vi "RW_Module.vi"(7 "N_moduls":i32, 8 "error in":errorcluster, 9 "Param Referense":T1, 10 "Data Reference":T2, 11 "Status Reference":T3) -> (0 "error out":errorcluster, 1 "stopped":bool)   [LabVIEW 2019]
uses:
  Eth Status/Ctl/ICPCON Status.ctl
  MB_TCP_State.ctl
  ICPCON Registers/Ctl/ICPCON Data.ctl
  ICPCON Param/ICPCON Param.ctl
  ICPCON Param/Eth timeouts.ctl
  ICPCON ET-7018/ICPCON ET-7018.lvclass
  D:/my_projects/projects/Algorithms/Labview/19/Modbus/MB_TCP2/MB_TCP.lvclass
  ICPCON ET-7016/ICPCON ET-7016.lvclass
  ICPCON ET-7051/ICPCON ET-7051.lvclass
  ICPCON ET-7017/ICPCON ET-7017.lvclass
  ICPCON ET-7018i/ICPCON ET-7018i.lvclass
  ICPCON ET-7024i/ICPCON ET-7024i.lvclass
  ZERO/ZERO.lvclass
  NS300/NS300.lvclass
  ICPCON ET-7042i/ICPCON ET-7042i.lvclass
  TEST/TEST.lvclass
  LIR-919D/LIR-919D.lvclass
  ICPCON ET-7016i/ICPCON ET-7016i.lvclass
  ICPCON ET-7024/ICPCON ET-7024.lvclass
  SMSD/SMSD-AI/SMSD-AI.lvclass
  SMSD/SMSD-DI/SMSD-DI.lvclass
  MB timeouts.ctl
  NI_modbus_upd/TCP/tcp timeouts.ctl
  MB_TCP.lvclass/MB_TCP.ctl
  NI_modbus_upd/TCP/TCP.lvclass/TCP.ctl
  Execute.vi
  MB_TCP.lvclass
  Eth Status/Eth Status.lvlib
  ICPCON Param/ICPCON_Param.lvlib
  NI_modbus_upd/TCP/TCP.lvclass
  ICPCON Registers/ICPCON Registers.lvlib
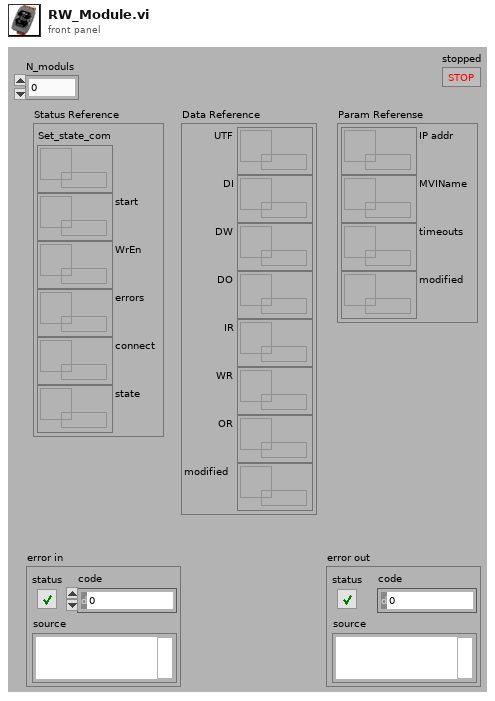
[diagram p1: front panel]
types:
  T1 = typedef "ICPCON_Param.lvlib/ICPCON Param.ctl" = cluster{"IP addr":refnum<data-value>, "MVIName":refnum<data-value>, "timeouts":refnum<data-value>, "modified":refnum<data-value>}
  T2 = typedef "ICPCON Registers.lvlib/ICPCON Data.ctl" = cluster{"UTF":refnum<data-value>, "DI":refnum<data-value>, "DW":refnum<data-value>, "DO":refnum<data-value>, "IR":refnum<data-value>, "WR":refnum<data-value>, "OR":refnum<data-value>, "modified":refnum<data-value>}
  T3 = typedef "Eth Status.lvlib/ICPCON Status.ctl" = cluster{"Set_state_com":refnum<data-value>, "start":refnum<data-value>, "WrEn":refnum<data-value>, "errors":refnum<data-value>, "connect":refnum<data-value>, "state":refnum<data-value>}
  T4 = enum16{"initialize", "call modules", "work", "stop modules", "standby"}
  T5 = typedef "TCP.lvclass/tcp timeouts.ctl" = cluster{"connect timeout":i32, "write timeout":i32, "read timeout":i32}
  T6 = typedef "MB_TCP.lvclass/MB timeouts.ctl" = cluster{"reconn_timeout":i32, "N attempt max":i32, "t_reset_TTL":i32, "period":i32}
  T7 = typedef "ICPCON_Param.lvlib/Eth timeouts.ctl" = cluster{"conn_timeout":i32, "reconn_timeout":i32, "N attempt max":i32, "t_reset_TTL":i32, "write_timeout":i32, "read_timeout":i32, "period":i32}
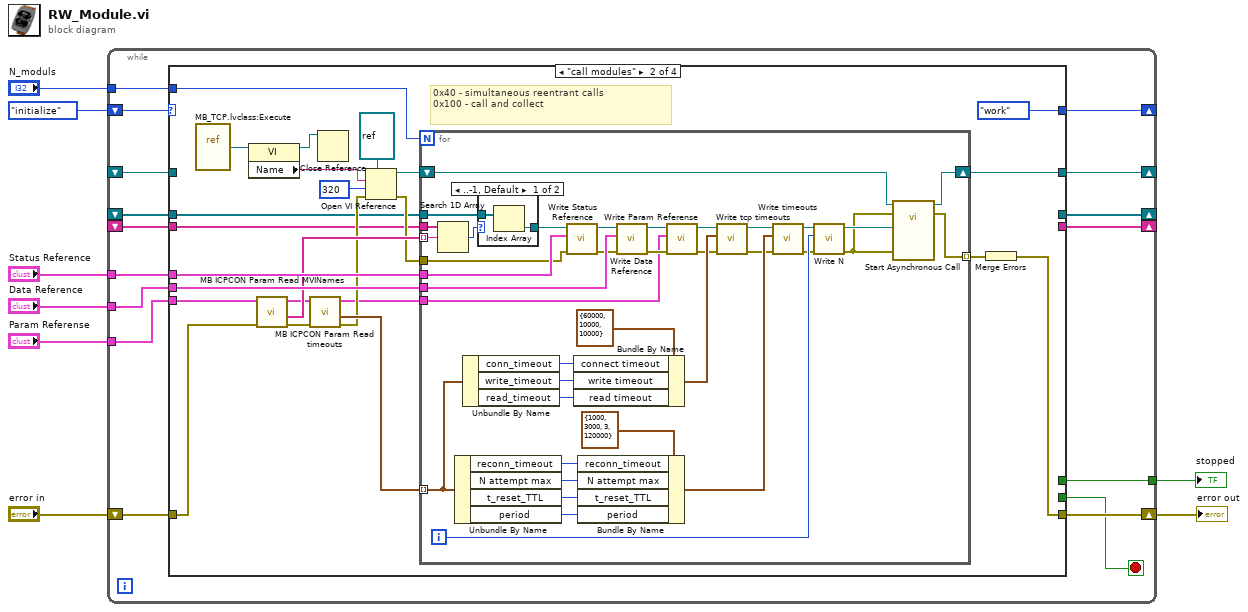
[diagram p0: block diagram]
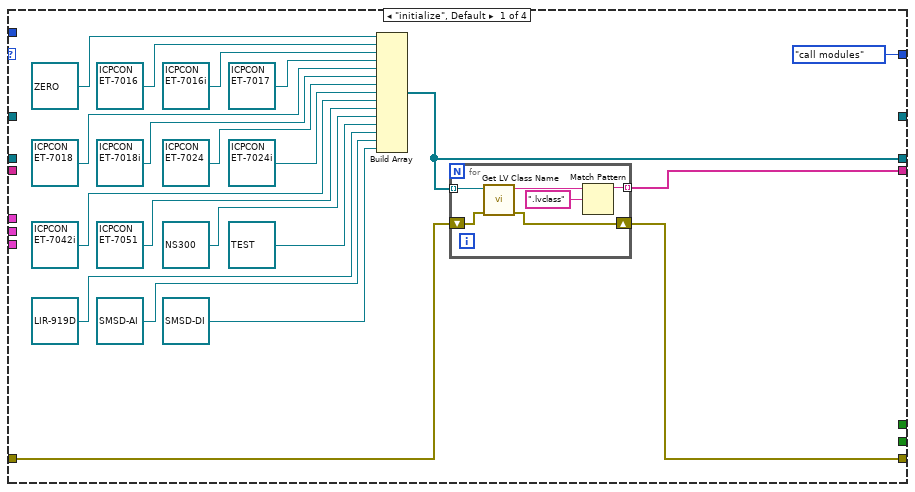
[diagram p2: hidden frame]
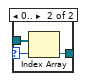
[diagram p3: hidden frame]
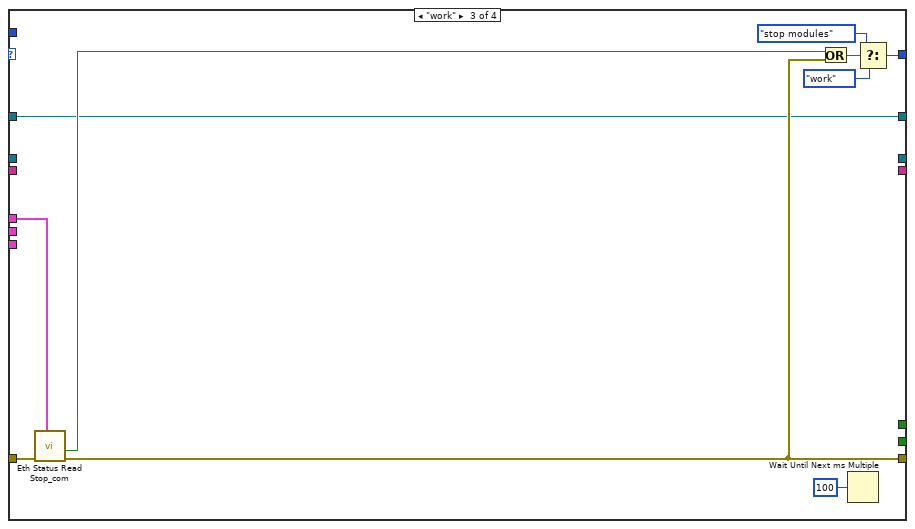
[diagram p4: hidden frame]
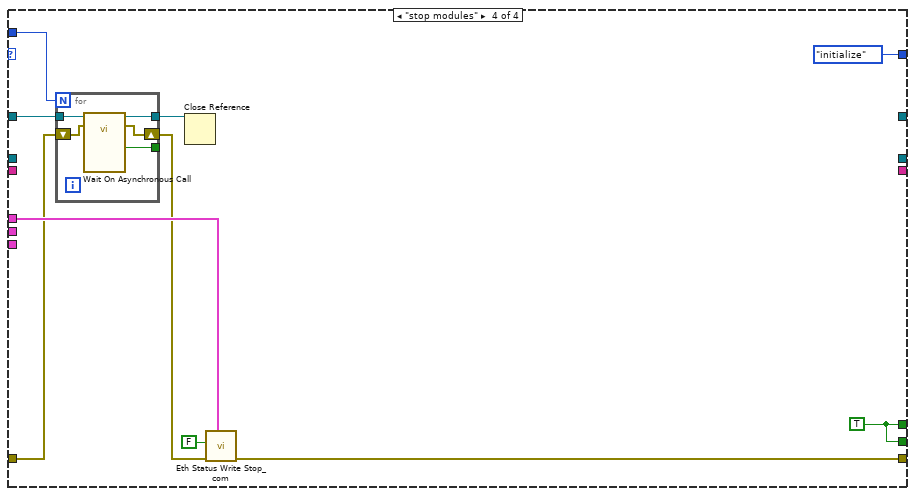
[diagram p5: hidden frame]
diagram:
  n1 = while {
    shift-right: [w24] -> _
    shift-left: T4."initialize" ("Enum") -> [w23]
    shift-right: [w22] -> w7
    shift-left: "error in" -> [w21]
    tunnel: [w20] -> w6
    tunnel: "Param Referense" -> [w18]
    tunnel: "Data Reference" -> [w17]
    tunnel: "Status Reference" -> [w16]
    tunnel: "N_moduls" -> [w15]
    shift-right: [w14] -> _
    shift-left: _ -> [w13]
    shift-right: [w12] -> _
    shift-left: _ -> [w10]
    shift-right: [w11] -> _
    shift-left: _ -> [w9]
    stop <- w19 stop-if-true
    n2 = case shown="\"call modules\"" w23 {
      tunnel: [T4."call modules" ("Enum") T4."work" ("Enum") w126 T4."initialize" ("Enum")] -> w24
      tunnel: w15 -> [_ w66 _ w127]
      tunnel: w16 -> [_ w73 w120 w134]
      tunnel: [w42 w72 w118 w133] -> w22
      tunnel: w21 -> [w43 w54 w121 w130]
      tunnel: [_ _ _ w136] -> w20
      tunnel: [_ _ _ w136] -> w19
      tunnel: w17 -> [_ w69 _ _]
      tunnel: w18 -> [_ w53 _ _]
      tunnel: [_ w57 w117 _] -> w14
      tunnel: w13 -> [_ _ w117 w131]
      tunnel: [w41 _ _ _] -> w12
      tunnel: [w40 _ _ _] -> w11
      tunnel: w10 -> [_ w56 _ _]
      tunnel: w9 -> [_ w55 _ _]
      frame "initialize", Default {
        n3 = Build Array(refnum<class "ZERO.lvclass"> refnum ("ZERO.lvclass"), refnum<class "ICPCON ET-7016.lvclass"> refnum ("ICPCON ET-7016.lvclass"), refnum<class "ICPCON ET-7016i.lvclass"> refnum ("ICPCON ET-7016i.lvclass"), refnum<class "ICPCON ET-7017.lvclass"> refnum ("ICPCON ET-7017.lvclass"), refnum<class "ICPCON ET-7018.lvclass"> refnum ("ICPCON ET-7018 in"), refnum<class "ICPCON ET-7018i.lvclass"> refnum ("ICPCON ET-7018i.lvclass"), refnum<class "ICPCON ET-7024.lvclass"> refnum ("ICPCON ET-7024.lvclass"), refnum<class "ICPCON ET-7024i.lvclass"> refnum ("ICPCON ET-7024i.lvclass"), refnum<class "ICPCON ET-7042i.lvclass"> refnum ("ICPCON ET-7042i.lvclass"), refnum<class "ICPCON ET-7051.lvclass"> refnum ("ICPCON ET-7051.lvclass"), refnum<class "NS300.lvclass"> refnum ("NS300.lvclass"), refnum<class "TEST.lvclass"> refnum ("TEST.lvclass"), refnum<class "LIR-919D.lvclass"> refnum ("LIR-919D.lvclass"), refnum<class "SMSD-AI.lvclass"> refnum ("SMSD-AI.lvclass"), refnum<class "SMSD-DI.lvclass"> refnum ("SMSD-DI.lvclass")) -> (w41:refnum<class "MB_TCP.lvclass">[])
        n4 = for {
          tunnel: w41 -> [w50] mode=indexing
          tunnel: [w46] -> w40 mode=indexing
          shift-right: [w49] -> w42
          shift-left: w43 -> [w45]
          n5 = call <vilib>:"Get LV Class Name.vi"("error in (no error)"=w45, "object"=w50) -> ("error out"=w49:errorcluster, "class name"=w48:string)  [unwired: 8 in]
          n6 = Match Pattern(string=w48, regular expression=".lvclass") -> (before substring=w46:string)  [unwired: 1 in, 3 out]
        }
      }
      frame "call modules" {
        # "0x40 - simultaneous reentrant calls\n0x100 - call and collect"
        n7 = vi-ref "MB_TCP.lvclass:Execute.vi"() -> (w70:refnum<vi>)
        n8 = property class="VI"(reference=w70) -> (reference out=w64:refnum<vi>, "Name"=w61:string)  [unwired: 1 in, 1 out]
        n9 = call "MB ICPCON Param Read MVINames.vi"("error in (no error)"=w54, "Param Reference in"=w53) -> ("error out"=w65:errorcluster, "MVIName"=w67:string[], "Param Reference out"=w52:T1)  [unwired: 7 in]
        n10 = call "MB ICPCON Param Read timeouts.vi"("error in (no error)"=w65, "Param Reference in"=w52) -> ("error out"=w62:errorcluster, "timeouts"=w68:T7[], "Param Reference out"=w51:T1)  [unwired: 7 in]
        n11 = Close Reference(reference=w64) -> ()  [unwired: 1 in, 1 out]
        n12 = Open VI Reference(type specifier VI Refnum (for type only)=refnum<vi> refnum, vi path=w61, options=320, error in (no error)=w62) -> (vi reference=w59:refnum<vi>, error out=w60:errorcluster)  [unwired: 2 in]
        n13 = for {
          N: w66 -> [_]
          tunnel: [w111] -> w74 mode=indexing
          tunnel: w68 -> [w81] mode=indexing
          tunnel: w67 -> [w97] mode=indexing
          tunnel: w73 -> [w108]
          tunnel: w69 -> [w107]
          tunnel: w56 -> [w110]
          tunnel: w55 -> [w109]
          tunnel: w60 -> [w96]
          shift-right: [w94] -> w57
          shift-left: w59 -> [w95]
          tunnel: w51 -> [w86]
          i -> [w99]
          n14 = Search 1D Array(1D array=w109, element=w97) -> (index of element=w106:i32)  [unwired: 1 in]
          n15 = Unbundle By Name(w81) -> ("reconn_timeout"=w104:i32, "N attempt max"=w103:i32, "t_reset_TTL"=w102:i32, "period"=w101:i32)
          n16 = Unbundle By Name(w81) -> ("conn_timeout"=w84:i32, "write_timeout"=w83:i32, "read_timeout"=w82:i32)
          n17 = case shown="..-1, Default" w106 {
            selector: w106 -> [_ w114]
            tunnel: w110 -> [w113 w116]
            tunnel: [w112 w115] -> w98
            frame ..-1, Default {
              n18 = Index Array(array=w113) -> (element=w112:refnum<class "MB_TCP.lvclass">)  [unwired: 1 in]
            }
            frame 0.. {
              n19 = Index Array(array=w116, index=w114) -> (element=w115:refnum<class "MB_TCP.lvclass">)
            }
          }
          n20 = call "Write Status Reference.vi"("error in (no error)"=w96, "Status"=w108, "MB_TCP in"=w98) -> ("error out"=w89:errorcluster, "MB_TCP out"=w90:refnum<class "MB_TCP.lvclass">)  [unwired: 7 in]
          n21 = Bundle By Name(cluster=T5 {"connect timeout"=60000, "write timeout"=10000, "read timeout"=10000} ("tcp timeouts"), "connect timeout"=w84, "write timeout"=w83, "read timeout"=w82) -> (w80:T5)
          n22 = Bundle By Name(cluster=T6 {"reconn_timeout"=1000, "N attempt max"=3000, "t_reset_TTL"=3, "period"=120000} ("timeouts"), "reconn_timeout"=w104, "N attempt max"=w103, "t_reset_TTL"=w102, "period"=w101) -> (w100:T6)
          n23 = call "Write Data Reference.vi"("error in (no error)"=w89, "Data"=w107, "MB_TCP in"=w90) -> ("error out"=w87:errorcluster, "MB_TCP out"=w88:refnum<class "MB_TCP.lvclass">)  [unwired: 7 in]
          n24 = call "Write Param Referense.vi"("error in (no error)"=w87, "Param Referense"=w86, "MB_TCP in"=w88) -> ("error out"=w78:errorcluster, "MB_TCP out"=w79:refnum<class "MB_TCP.lvclass">)  [unwired: 7 in]
          n25 = call "Write tcp timeouts.vi"("error in (no error)"=w78, "tcp timeouts"=w80, "MB_TCP in"=w79) -> ("error out"=w76:errorcluster, "MB_TCP out"=w77:refnum<class "MB_TCP.lvclass">)  [unwired: 7 in]
          n26 = call "Write timeouts.vi"("error in (no error)"=w76, "MB timeouts"=w100, "MB_TCP in"=w77) -> ("error out"=w92:errorcluster, "MB_TCP out"=w91:refnum<class "MB_TCP.lvclass">)  [unwired: 7 in]
          n27 = call "Write N.vi"("error in (no error)"=w92, "N"=w99, "MB_TCP in"=w91) -> ("error out"=w75:errorcluster, "MB_TCP out"=w93:refnum<class "MB_TCP.lvclass">)  [unwired: 7 in]
          n28 = call-by-ref "Start Asynchronous Call"(reference=w95, error in=w75, 8:"error in (no error)"=w75, "MB_TCP in"=w93) -> (reference out=w94:refnum<vi>, error out=w111:errorcluster)  [unwired: 7 in, 3 out]
        }
        n29 = Merge Errors(w74) -> (w72:errorcluster)
      }
      frame "work" {
        n30 = call "Eth Status Read Stop_com.vi"("Status Reference"=w120, "error in (no error)"=w121) -> ("error out"=w118:errorcluster, "Stop"=w119:bool)  [unwired: 8 in]
        n31 = Or(x=w119, y=w118) -> (x .or. y?=w125:bool)
        n32 = Wait Until Next ms Multiple(millisecond multiple=u32 100) -> ()  [unwired: 1 out]
        n33 = Select(t=T4."stop modules" ("Enum"), s=w125, f=T4."work" ("Enum")) -> (s? t:f=w126:T4)
      }
      frame "stop modules" {
        w136 = TRUE
        n34 = for {
          N: w127 -> [_]
          tunnel: w131 -> [w141]
          tunnel: [w139] -> w129
          shift-right: [w138] -> w128
          shift-left: w130 -> [w140]
          tunnel: [w137] -> _
          n35 = call-by-ref "Wait On Asynchronous Call"(reference=w141, error in=w140) -> (reference out=w139:refnum<vi>, error out=w138:errorcluster, "stopped"=w137:bool)  [unwired: 9 in, 2 out]
        }
        n36 = Close Reference(reference=w129) -> ()  [unwired: 1 in, 1 out]
        n37 = call "Eth Status Write Stop_com.vi"("Status Reference"=w134, "error in (no error)"=w128, "Stop"=FALSE) -> ("error out"=w133:errorcluster)  [unwired: 8 in]
      }
    }
  }
  "error out" <- w7
  "stopped" <- w6
